vi "Home.vi"(8 "error in (no error)":errorcluster, 11 "Character LCD in":refnum<class "Grove I2C LCD.lvclass">) -> (0 "error out":errorcluster, 3 "Character LCD out":refnum<class "Grove I2C LCD.lvclass">)   [LabVIEW 2020, in "CTI-Peripheral.lvlib" / "Grove I2C LCD.lvclass"]
uses:
  Grove I2C LCD.lvclass
  Grove I2C LCD.lvclass/Grove I2C LCD.ctl
  HD44780 LCD/Command.ctl
  HD44780 LCD/HD44780 LCD.lvlib
  348a0649-b16d-4b51-9571-44a0d633c5f2.vi
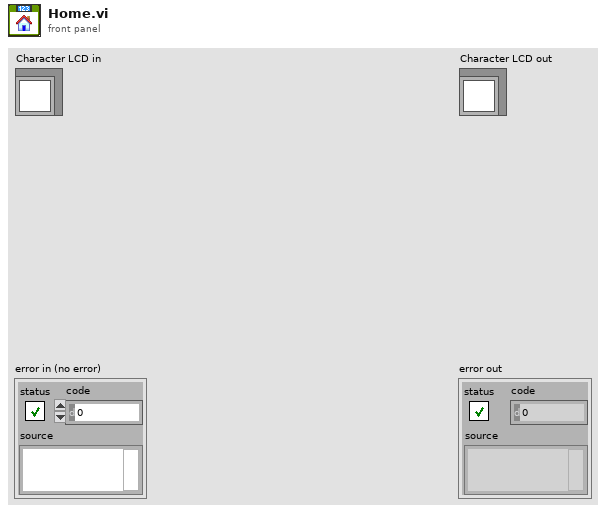
[diagram p1: front panel]
types:
  T1 = typedef "CTI-Peripheral.lvlib/HD44780 LCD.lvlib/Command.ctl" = enum16{"ClearDisplay", "ReturnHome", "EntryModeSet", "DisplayControl", "CursorShift", "FunctionSet", "SetCGRamAddr", "SetDDRamAddr"}
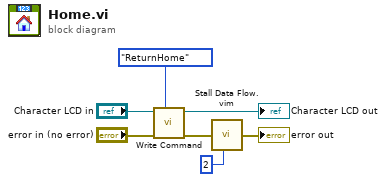
[diagram p0: block diagram]
diagram:
  n1 = call "Write Command.vi"("Command"=Command."ReturnHome", "error in (no error)"="error in (no error)", "Grove I2C LCD in"="Character LCD in") -> ("error out"=w6:errorcluster, "Grove I2C LCD out"=→"Character LCD out":refnum<class "Grove I2C LCD.lvclass">)  [unwired: 7 in]
  n2 = call "Stall Data Flow.vim"("value in"=w6, "milliseconds to wait"=u32 2) -> ("value out"=→"error out":errorcluster)  [unwired: 1 out]
